vi "Write Charm SubPanel.vi"(8 "error in (no error)":errorcluster, 10 "Charm SubPanel":refnum<vi>, 11 "MainController in":refnum<class "MainController.lvclass">) -> (0 "error out":errorcluster, 3 "MainController out":refnum<class "MainController.lvclass">)   [LabVIEW 2020, in "MainController.lvlib" / "MainController.lvclass"]
uses:
  MainController.lvclass
  MainController.lvclass/MainController.ctl
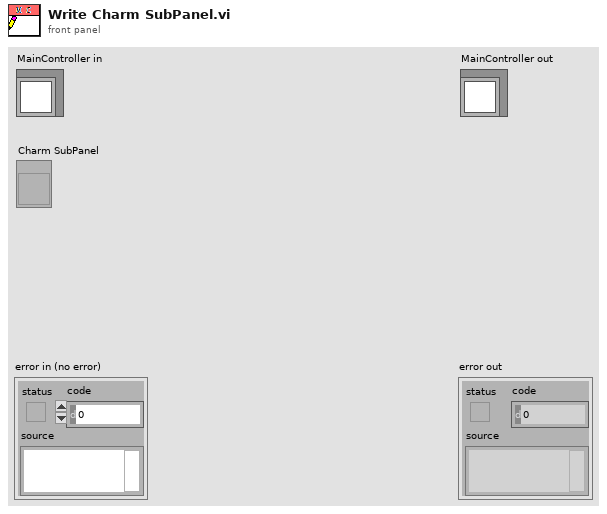
[diagram p1: front panel]
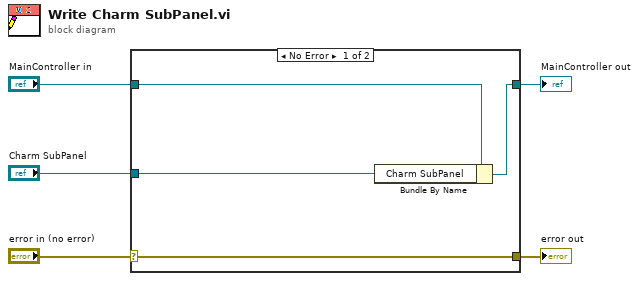
[diagram p0: block diagram]
diagram:
  n1 = case shown="No Error" "error in (no error)" {
    selector: "error in (no error)" -> [w9 w10]
    tunnel: [w9 w10] -> w4
    tunnel: [w7 w11] -> w2
    tunnel: "MainController in" -> [w8 w11]
    tunnel: "Charm SubPanel" -> [w6 _]
    frame No Error {
      n2 = Bundle By Name(cluster=w8, "Charm SubPanel"=w6) -> (w7:refnum<class "MainController.lvclass">)
    }
    frame Error {
    }
  }
  "error out" <- w4
  "MainController out" <- w2
